vi "Add Actor.vi"(8 "error in":errorcluster, 11 "Target Item":T1) -> (0 "error out":errorcluster)   [LabVIEW 2020, in "Add Actor.lvlib"]
uses:
  Add Actor.lvlib
  Localized Strings.vi
  Classes/INI Store/INI Store.lvclass
  Classes/Target Store/Target Store.lvclass
  MessageMakerProvider/AFPP Shared/AFPP Shared.lvlib
  <resource>/Framework/Providers/API/mxLvNIIM.ctl
panel:
  out "Path Display":string
  in  "Path":path caption="Save files to..."
  in  "Remove Actor":bool
  in  "Inherit from:":string(combo)
  in  "Cancel Button":bool
  in  "OK Button":bool
  in  "Name of Actor":string
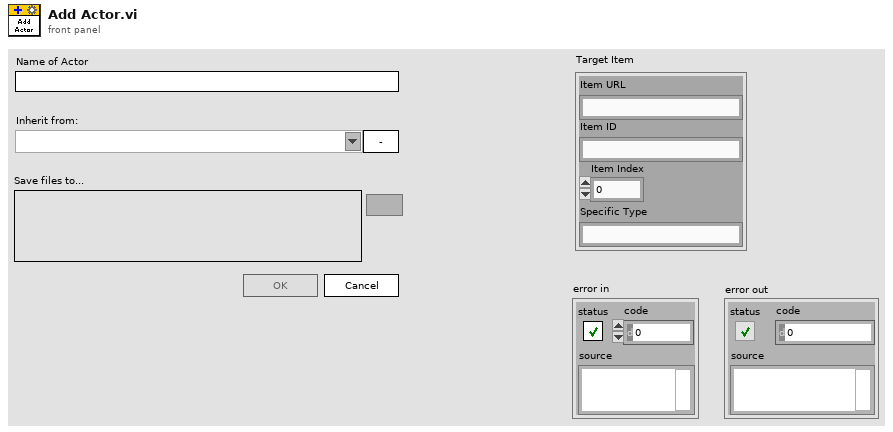
[diagram p1: front panel]
types:
  T1 = typedef "mxLvNIIM.ctl" = cluster{"Item URL":string, "Item ID":string, "Item Index":i32, "Specific Type":string}
  T2 = enum8{"Enabled", "Disabled", "Disabled and Grayed Out"}
  T3 = enum32{"Invalid", "Standard", "Closed", "Hidden", "Minimized", "Maximized"}
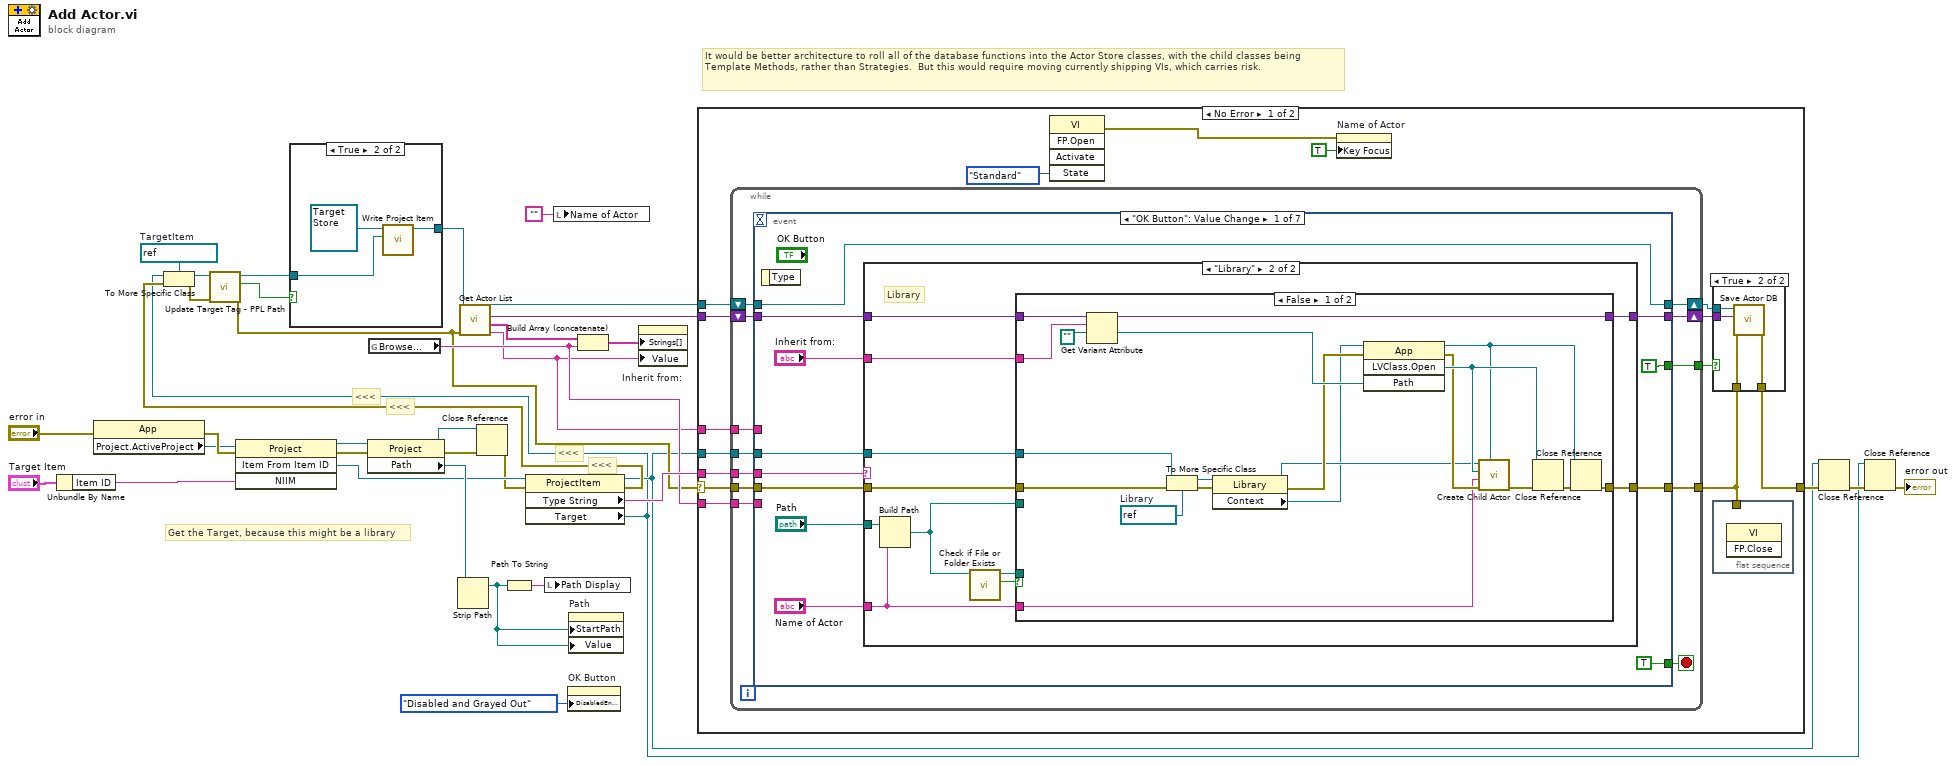
[diagram p0: block diagram]
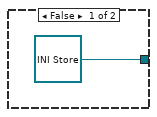
[diagram p2: hidden frame]
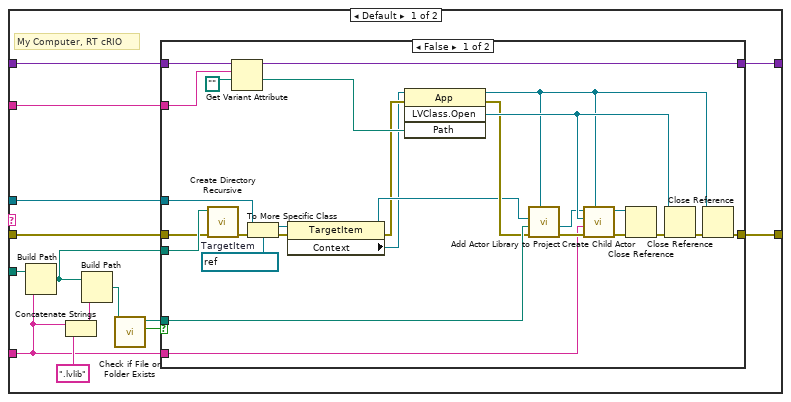
[diagram p3: hidden frame]
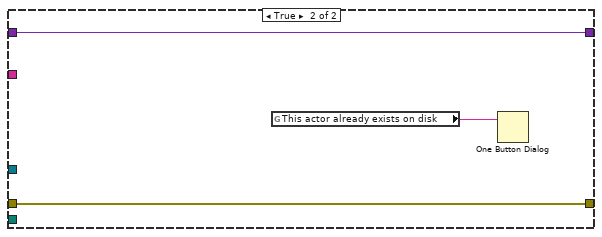
[diagram p4: hidden frame]
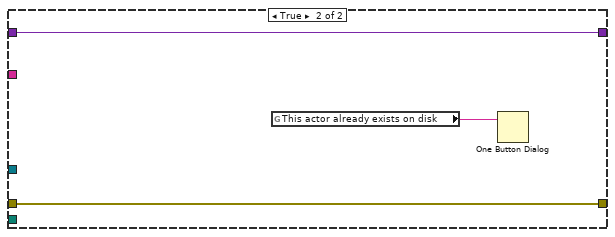
[diagram p5: hidden frame]
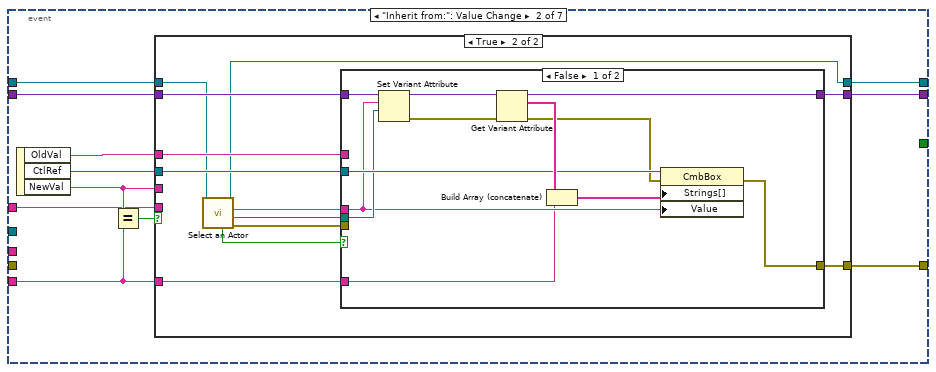
[diagram p6: hidden frame]
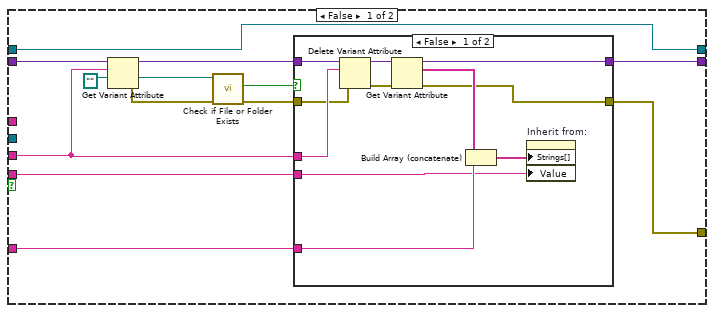
[diagram p7: hidden frame]
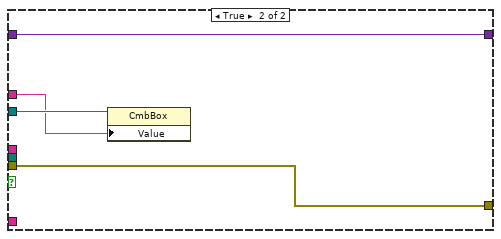
[diagram p9: hidden frame]
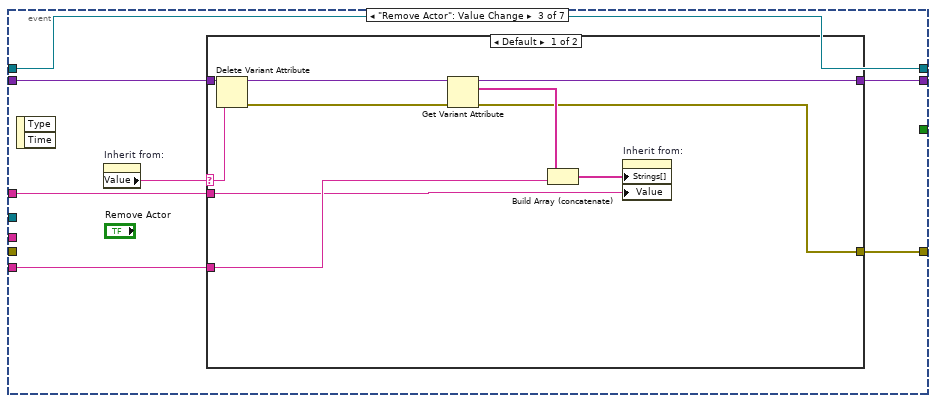
[diagram p10: hidden frame]
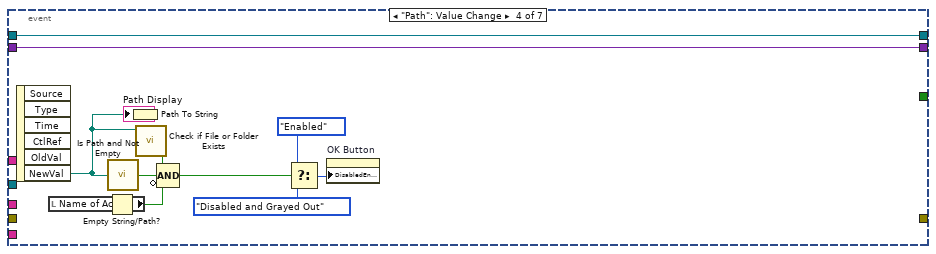
[diagram p12: hidden frame]
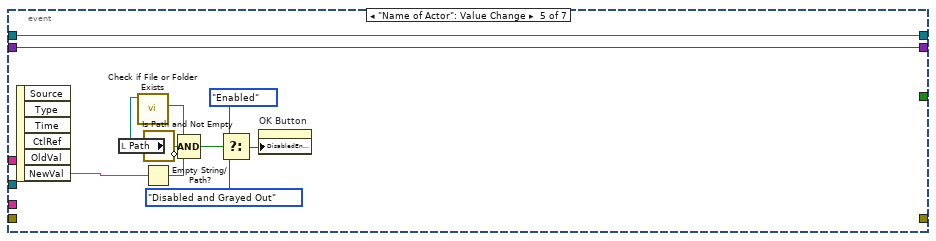
[diagram p13: hidden frame]
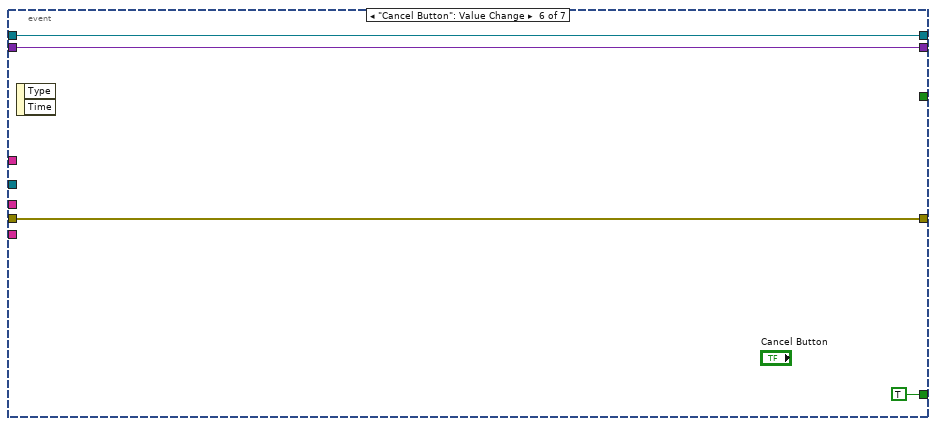
[diagram p14: hidden frame]
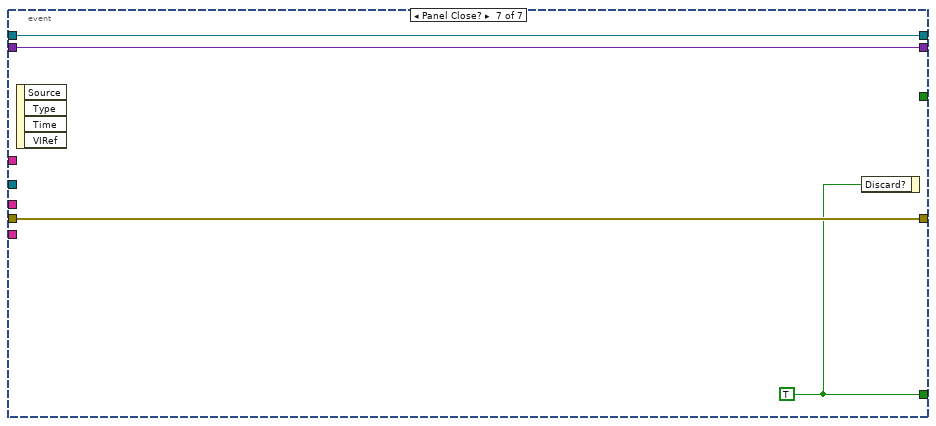
[diagram p15: hidden frame]
diagram:
  w7 = refnum<vi> refnum  # TargetItem
  # "Get the Target, because this might be a library"
  # "<<<"
  # "<<<"
  # "<<<"
  # "<<<"
  # "It would be better architecture to roll all of the database functions into the Actor Store classes, with the child classes being Template Methods, rather than Strategies.  But this would require moving currently shipping VIs, which carries risk."
  n1 = Unbundle By Name("Target Item") -> ("Item ID"=w30:string)
  n2 = property class="App"(error in="error in") -> (error out=w34:errorcluster, "Project.ActiveProject"=w33:refnum<vi>)  [unwired: 1 in, 1 out]
  n3 = invoke class="Project" method="Item From Item ID"(reference=w33, error in=w34, "NIIM"=w30) -> (reference out=w26:refnum<vi>, error out=w27:errorcluster, "GetItemFromNIIM"=w22:refnum<vi>)  [unwired: 1 in, 1 out]
  n4 = property class="Project"(reference=w26, error in=w27) -> (reference out=w16:refnum<vi>, error out=w18:errorcluster, "Path"=w29:path)
  n5 = global read "Localized Strings.vi" "Browse..."() -> (w23:string)
  n6 = Strip Path(path=w29) -> (stripped path=w20:path)  [unwired: 1 out]
  n7 = Close Reference(reference=w16, error in (no error)=w18) -> (error out=w17:errorcluster)
  n8 = Path To String(path=w20) -> (string=w21:string)
  n9 = property class="ProjectItem"(reference=w22, error in=w17) -> (reference out=w2:refnum<vi>, error out=w4:errorcluster, "Type String"=w28:string, "Target"=w1:refnum<vi>)
  n10 = To More Specific Class(target class=w7, reference=w1, error in=w4) -> (specific class reference=w6:refnum<vi>, error out=w5:errorcluster)
  n11 = call "Update Target Tag - PPL Path.vi"("error in (no error)"=w5, "Target"=w6) -> ("error out"=w8:errorcluster, "Found PPL?"=w15:bool, "dup Target"=w13:refnum<vi>)  [unwired: 7 in]
  n12 = case shown="True" w15 {
    tunnel: [refnum<class "INI Store.lvclass"> refnum ("Add Actor.lvlib:INI Store.lvclass") w40] -> w14
    tunnel: w13 -> [_ w38]
    frame False {
    }
    frame True {
      n13 = call-dynamic "Write Project Item.vi"("Project Item"=w38, "Target Store in"=refnum<class "Target Store.lvclass"> refnum) -> ("Target Store out"=w40:refnum<class "Target Store.lvclass">)  [unwired: 9 in]
    }
  }
  n14 = call "Get Actor List.vi"("error in (no error)"=w8, "Actor Store"=w14) -> ("Actor Label"=w19:string, "Actors"=w11:string[], "Actor Paths"=w36:variant, "Actor Store"=w12:refnum<class "Actor Store.lvclass">)  [unwired: 6 in]
  n15 = local write "Path Display"(w21) -> ()
  n16 = local write "Name of Actor"("" ("Name of Actor")) -> ()
  n17 = property on="OK Button" class="Bool"("DisabledEnum"=T2."Disabled and Grayed Out" ("Disabled")) -> ()  [unwired: 2 in, 2 out]
  n18 = property on="Path" class="Path"("StartPath"=w20, "Value"=w20) -> ()  [unwired: 2 in, 2 out]
  n19 = Build Array (concatenate)(w11, w23) -> (w35:string[])
  n20 = property on="Inherit from:" class="CmbBox"("Strings[]"=w35, "Value"=w19) -> ()  [unwired: 2 in, 2 out]
  n21 = case shown="No Error" w8 {
    selector: w8 -> [w55 w277]
    tunnel: [w49 w277] -> w9
    tunnel: w36 -> [w54 _]
    tunnel: w28 -> [w53 _]
    tunnel: w2 -> [w52 _]
    tunnel: w23 -> [w51 _]
    tunnel: w19 -> [w47 _]
    tunnel: w12 -> [w46 _]
    frame No Error {
      n22 = while {
        tunnel: [w67] -> w43
        tunnel: w55 -> [w66]
        shift-right: [w63] -> w50
        shift-left: w54 -> [w64]
        tunnel: w53 -> [w62]
        tunnel: w52 -> [w61]
        tunnel: w51 -> [w60]
        tunnel: [w59] -> w48
        tunnel: w47 -> [w58]
        shift-right: [w56] -> w45
        shift-left: w46 -> [w57]
        stop <- w65 stop-if-true
        n23 = event shown="[0] \"OK Button\": Value Change" {
          selector: _ -> [_ _ _ _ _ _ _]
          dyn-events: _ -> [_ _ _ _ _ _ _]
          timeout: _ -> [_ _ _ _ _ _ _]
          tunnel: w66 -> [w73 _ _ _ _ w266 w271]
          tunnel: [w74 w168 w226 _ _ w266 w271] -> w67
          tunnel: [TRUE _ _ _ _ TRUE w269] -> w65
          tunnel: w64 -> [w77 w167 w228 w249 w256 w265 w270]
          tunnel: [w75 w166 w227 w249 w256 w265 w270] -> w63
          tunnel: w62 -> [w72 _ _ _ _ _ _]
          tunnel: w61 -> [w71 _ _ _ _ _ _]
          tunnel: w60 -> [_ w162 w225 _ _ _ _]
          tunnel: [TRUE _ _ _ _ _ _] -> w59
          tunnel: w58 -> [_ w161 w224 _ _ _ _]
          tunnel: w57 -> [w68 w159 w223 w241 w253 w264 w268]
          tunnel: [w68 w158 w223 w241 w253 w264 w268] -> w56
          event "OK Button": Value Change {
            n24 = event-data() -> ()  [unwired: 1 in, 1 out]
            n25 = case shown="\"Library\"" w72 {
              tunnel: "Path" -> [w93 w134]
              tunnel: "Name of Actor" -> [w81 w125]
              tunnel: w77 -> [w92 w133]
              tunnel: "Inherit from:" -> [w91 w132]
              tunnel: [w90 w131] -> w75
              tunnel: [w87 w129] -> w74
              tunnel: w73 -> [w86 w128]
              tunnel: w71 -> [w84 w126]
              frame Default {
                # "My Computer, RT cRIO"
                n26 = Build Path(base path=w93, name or relative path=w81) -> (appended path=w89:path)
                n27 = Concatenate Strings(w81, ".lvlib" ("string")) -> (w82:string)
                n28 = Build Path(base path=w89, name or relative path=w82) -> (appended path=w80:path)
                n29 = call <vilib>:"Check if File or Folder Exists.vi"("path"=w80) -> ("file or folder exists?"=w85:bool, "dup path"=w88:path)  [unwired: 8 in, 1 out]
                n30 = case shown="False" w85 {
                  tunnel: w81 -> [w104 _]
                  tunnel: w92 -> [w119 w123]
                  tunnel: w91 -> [w118 _]
                  tunnel: [w117 w123] -> w90
                  tunnel: w89 -> [w103 _]
                  tunnel: w88 -> [w114 _]
                  tunnel: [w105 w122] -> w87
                  tunnel: w86 -> [w102 w122]
                  tunnel: w84 -> [w108 _]
                  frame False {
                    w113 = refnum<vi> refnum  # TargetItem
                    n31 = call <vilib>:"Create Directory Recursive.vi"("error in (no error)"=w102, "directory"=w103) -> ("error out"=w101:errorcluster)  [unwired: 3 in, 2 out]
                    n32 = Get Variant Attribute(Variant=w119, name=w118, default value (empty Variant)=path "") -> (duplicate Variant=w117:variant, value=w116:path)  [unwired: 1 in, 2 out]
                    n33 = To More Specific Class(target class=w113, reference=w108, error in=w101) -> (specific class reference=w100:refnum<vi>, error out=w98:errorcluster)
                    n34 = property class="TargetItem"(reference=w100, error in=w98) -> (reference out=w99:refnum<vi>, error out=w97:errorcluster, "Context"=w96:refnum<vi>)
                    n35 = invoke class="App" method="LVClass.Open"(reference=w96, error in=w97, "Path"=w116) -> (reference out=w95:refnum<vi>, error out=w107:errorcluster, "LVClass.Open"=w120:refnum<vi>)  [unwired: 1 in, 1 out]
                    n36 = call "Add Actor Library to Project.vi"("Application"=w95, "error in (no error)"=w107, "Library Path"=w114, "Target Item"=w99) -> ("error out"=w112:errorcluster, "Library out"=w111:refnum<vi>)  [unwired: 6 in]
                    n37 = call "Create Child Actor.vi"("App Inst"=w95, "error in (no error)"=w112, "Actor Name"=w104, "Parent Class"=w120, "Library in"=w111) -> ("error out"=w110:errorcluster, "Library out"=w109:refnum<vi>)  [unwired: 5 in]
                    n38 = Close Reference(reference=w109, error in (no error)=w110) -> (error out=w94:errorcluster)
                    n39 = Close Reference(reference=w120, error in (no error)=w94) -> (error out=w106:errorcluster)
                    n40 = Close Reference(reference=w95, error in (no error)=w106) -> (error out=w105:errorcluster)
                  }
                  frame True {
                    n41 = global read "Localized Strings.vi" "This actor already exists on disk"() -> (w121:string)
                    n42 = One Button Dialog(message=w121) -> ()  [unwired: 1 in, 1 out]
                  }
                }
              }
              frame "Library" {
                # "Library"
                n43 = Build Path(base path=w134, name or relative path=w125) -> (appended path=w124:path)
                n44 = call <vilib>:"Check if File or Folder Exists.vi"("path"=w124) -> ("file or folder exists?"=w127:bool, "dup path"=w130:path)  [unwired: 8 in, 1 out]
                n45 = case shown="False" w127 {
                  tunnel: w125 -> [w143 _]
                  tunnel: w133 -> [w153 w157]
                  tunnel: w132 -> [w152 _]
                  tunnel: [w151 w157] -> w131
                  tunnel: w124 -> [_ _]
                  tunnel: w130 -> [_ _]
                  tunnel: [w144 w156] -> w129
                  tunnel: w128 -> [w142 w156]
                  tunnel: w126 -> [w147 _]
                  frame False {
                    w148 = refnum<vi> refnum  # Library
                    n46 = Get Variant Attribute(Variant=w153, name=w152, default value (empty Variant)=path "") -> (duplicate Variant=w151:variant, value=w150:path)  [unwired: 1 in, 2 out]
                    n47 = To More Specific Class(target class=w148, reference=w147, error in=w142) -> (specific class reference=w140:refnum<vi>, error out=w138:errorcluster)
                    n48 = property class="Library"(reference=w140, error in=w138) -> (reference out=w139:refnum<vi>, error out=w141:errorcluster, "Context"=w137:refnum<vi>)
                    n49 = invoke class="App" method="LVClass.Open"(reference=w137, error in=w141, "Path"=w150) -> (reference out=w136:refnum<vi>, error out=w146:errorcluster, "LVClass.Open"=w154:refnum<vi>)  [unwired: 1 in, 1 out]
                    n50 = call "Create Child Actor.vi"("App Inst"=w136, "error in (no error)"=w146, "Actor Name"=w143, "Parent Class"=w154, "Library in"=w139) -> ("error out"=w135:errorcluster)  [unwired: 5 in, 1 out]
                    n51 = Close Reference(reference=w154, error in (no error)=w135) -> (error out=w145:errorcluster)
                    n52 = Close Reference(reference=w136, error in (no error)=w145) -> (error out=w144:errorcluster)
                  }
                  frame True {
                    n53 = global read "Localized Strings.vi" "This actor already exists on disk"() -> (w155:string)
                    n54 = One Button Dialog(message=w155) -> ()  [unwired: 1 in, 1 out]
                  }
                }
              }
            }
          }
          event "Inherit from:": Value Change {
            n55 = event-data() -> ("OldVal"=w160:string, "CtlRef"=w165:refnum<vi>, "NewVal"=w163:string)  [unwired: 1 in]
            n56 = Equal?(x=w163, y=w162) -> (x = y?=w164:bool)
            n57 = case shown="True" w164 {
              tunnel: [w174 w200] -> w168
              tunnel: w167 -> [w181 w202]
              tunnel: [w175 w201] -> w166
              tunnel: w165 -> [_ w199]
              tunnel: w163 -> [w172 _]
              tunnel: w162 -> [w171 w198]
              tunnel: w161 -> [w170 _]
              tunnel: w160 -> [_ w197]
              tunnel: w159 -> [w169 w196]
              tunnel: [w169 w195] -> w158
              frame False {
                n58 = Get Variant Attribute(Variant=w181, name=w172, default value (empty Variant)=path "") -> (duplicate Variant=w178:variant, value=w180:path, error out=w177:errorcluster)  [unwired: 1 in, 1 out]
                n59 = call <vilib>:"Check if File or Folder Exists.vi"("error in (no error)"=w177, "path"=w180) -> ("error out"=w176:errorcluster, "file or folder exists?"=w173:bool)  [unwired: 7 in, 1 out]
                n60 = case shown="False" w173 {
                  tunnel: w178 -> [w192 w194]
                  tunnel: w172 -> [w191 _]
                  tunnel: w176 -> [w190 w193]
                  tunnel: [w185 w194] -> w175
                  tunnel: [w184 w193] -> w174
                  tunnel: w171 -> [w183 _]
                  tunnel: w170 -> [w182 _]
                  frame False {
                    n61 = Delete Variant Attribute(4:w190, 6:w191, 7:w192) -> (0:w186:errorcluster, 3:w189:variant)  [unwired: 1 out]
                    n62 = Get Variant Attribute(Variant=w189, error in=w186) -> (duplicate Variant=w185:variant, names=w187:string[], error out=w184:errorcluster)  [unwired: 2 in, 1 out]
                    n63 = Build Array (concatenate)(w187, w183) -> (w188:string[])
                    n64 = property on="Inherit from:" class="CmbBox"("Strings[]"=w188, "Value"=w182) -> ()  [unwired: 2 in, 2 out]
                  }
                  frame True {
                  }
                }
              }
              frame True {
                n65 = call "Select an Actor.vi"("Actor Store"=w196) -> ("error out"=w206:errorcluster, "Path to Actor"=w205:path, "Name of Actor"=w204:string, "Actor Store"=w195:refnum<class "Actor Store.lvclass">, "Cancelled"=w203:bool)  [unwired: 6 in]
                n66 = case shown="False" w203 {
                  tunnel: w204 -> [w208 _]
                  tunnel: w205 -> [w210 _]
                  tunnel: w206 -> [_ w221]
                  tunnel: w202 -> [w212 w222]
                  tunnel: [w215 w222] -> w201
                  tunnel: [w213 w221] -> w200
                  tunnel: w199 -> [w217 w220]
                  tunnel: w198 -> [w207 _]
                  tunnel: w197 -> [_ w219]
                  frame False {
                    n67 = Set Variant Attribute(Variant=w212, name=w208, value=w210) -> (Variant out=w211:variant, error out=w209:errorcluster)  [unwired: 1 in, 1 out]
                    n68 = Get Variant Attribute(Variant=w211, error in=w209) -> (duplicate Variant=w215:variant, names=w218:string[], error out=w214:errorcluster)  [unwired: 2 in, 1 out]
                    n69 = Build Array (concatenate)(w218, w207) -> (w216:string[])
                    n70 = property class="CmbBox"(reference=w217, error in=w214, "Strings[]"=w216, "Value"=w208) -> (error out=w213:errorcluster)  [unwired: 1 out]
                  }
                  frame True {
                    n71 = property class="CmbBox"(reference=w220, "Value"=w219) -> ()  [unwired: 1 in, 2 out]
                  }
                }
              }
            }
          }
          event "Remove Actor": Value Change {
            n72 = event-data() -> ()  [unwired: 1 in, 2 out]
            n73 = property on="Inherit from:" class="CmbBox"() -> ("Value"=w229:string)  [unwired: 2 in, 2 out]
            n74 = case shown="Default" w229 {
              selector: w229 -> [w235 _]
              tunnel: w228 -> [w238 w240]
              tunnel: [w237 w240] -> w227
              tunnel: [w236 _] -> w226
              tunnel: w225 -> [w231 _]
              tunnel: w224 -> [w230 _]
              frame Default {
                n75 = Delete Variant Attribute(6:w235, 7:w238) -> (0:w232:errorcluster, 3:w233:variant)  [unwired: 1 in, 1 out]
                n76 = Get Variant Attribute(Variant=w233, error in=w232) -> (duplicate Variant=w237:variant, names=w239:string[], error out=w236:errorcluster)  [unwired: 2 in, 1 out]
                n77 = Build Array (concatenate)(w239, w231) -> (w234:string[])
                n78 = property on="Inherit from:" class="CmbBox"("Strings[]"=w234, "Value"=w230) -> ()  [unwired: 2 in, 2 out]
              }
              frame "Actor", "Browse..." {
              }
            }
          }
          event "Path": Value Change {
            n79 = event-data() -> ("NewVal"=w242:path)  [unwired: 1 in, 5 out]
            n80 = local read "Name of Actor"() -> (w248:string)
            n81 = Empty String/Path?(string/path=w248) -> (empty?=w247:bool)
            n82 = call <vilib>:"Is Path and Not Empty.vi"("path"=w242) -> ("Is Path and Not Empty?"=w246:bool)  [unwired: 4 in]
            n83 = Path To String(path=w242) -> (string=→"Path Display":string)
            n84 = call <vilib>:"Check if File or Folder Exists.vi"("path"=w242) -> ("file or folder exists?"=w243:bool)  [unwired: 8 in, 2 out]
            n85 = Compound Arithmetic op=AND(w243, w246, invert w247) -> (w245:bool)
            n86 = Select(t=T2."Enabled" ("Disabled"), s=w245, f=T2."Disabled and Grayed Out" ("Disabled")) -> (s? t:f=w251:T2)
            n87 = property on="OK Button" class="Bool"("DisabledEnum"=w251) -> ()  [unwired: 2 in, 2 out]
          }
          event "Name of Actor": Value Change {
            n88 = event-data() -> ("NewVal"=w257:string)  [unwired: 1 in, 5 out]
            n89 = local read "Path"() -> (w254:path)
            n90 = call <vilib>:"Check if File or Folder Exists.vi"("path"=w254) -> ("file or folder exists?"=w255:bool)  [unwired: 8 in, 2 out]
            n91 = Empty String/Path?(string/path=w257) -> (empty?=w260:bool)
            n92 = call <vilib>:"Is Path and Not Empty.vi"("path"=w254) -> ("Is Path and Not Empty?"=w259:bool)  [unwired: 4 in]
            n93 = Compound Arithmetic op=AND(w255, w259, invert w260) -> (w258:bool)
            n94 = Select(t=T2."Enabled" ("Disabled"), s=w258, f=T2."Disabled and Grayed Out" ("Disabled")) -> (s? t:f=w262:T2)
            n95 = property on="OK Button" class="Bool"("DisabledEnum"=w262) -> ()  [unwired: 2 in, 2 out]
          }
          event "Cancel Button": Value Change {
            n96 = event-data() -> ()  [unwired: 1 in, 2 out]
          }
          event Panel Close? {
            w269 = TRUE
            n97 = event-data() -> ()  [unwired: 1 in, 4 out]
            n98 = event-data("Discard?"=w269) -> ()  [unwired: 1 in, 1 out]
          }
        }
      }
      n99 = invoke class="VI" method="FP.Open"("State"=T3."Standard") -> (error out=w41:errorcluster)  [unwired: 4 in, 4 out]
      n100 = property on="Name of Actor" class="Str"(error in=w41, "Key Focus"=TRUE) -> ()  [unwired: 1 in, 2 out]
      n101 = case shown="True" w48 {
        tunnel: w50 -> [_ w274]
        tunnel: [w272 w276] -> w49
        tunnel: w43 -> [w272 w275]
        tunnel: w45 -> [_ w273]
        frame False {
        }
        frame True {
          n102 = call "Save Actor DB.vi"("error in (no error)"=w275, "Actor DB"=w274, "Actor Store"=w273) -> ("error out"=w276:errorcluster)  [unwired: 6 in, 2 out]
        }
      }
      n103 = flat-sequence {
        tunnel: w43 -> [_]
        frame #0 {
          n104 = invoke class="VI" method="FP.Close"() -> ()  [unwired: 3 in, 3 out]
        }
      }
    }
    frame Error {
    }
  }
  n105 = Close Reference(reference=w2, error in (no error)=w9) -> (error out=w10:errorcluster)
  n106 = Close Reference(reference=w1, error in (no error)=w10) -> (error out=→"error out":errorcluster)
